vi "graficos3.vi"() -> ()   [LabVIEW 2019]
panel:
  out "Waveform Graph 3":cluster{dbl[]}[](graph)
  out "Waveform Graph 2":cluster{dbl, dbl, dbl[]}(graph)
  out "Waveform Chart 4":waveform(dbl)(graph)
  out "Waveform Chart 3":cluster{dbl, "Slide":dbl}(graph)
  out "Waveform Chart 2":dbl[](graph)
  out "Waveform Graph":dbl[](graph)
  out "Waveform Chart":dbl(graph)
  in  "stop":bool
  in  "Slide":dbl(slide) scale=0.0..50.0
  out "Thermometer":dbl(slide) scale=0.0..50.0
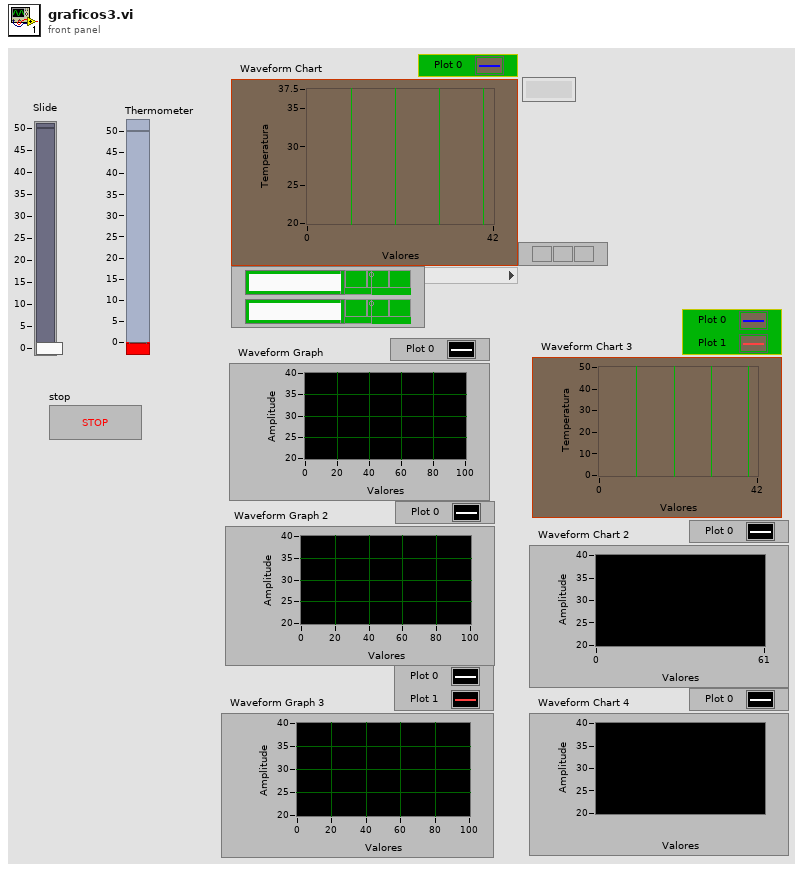
[diagram p1: front panel]
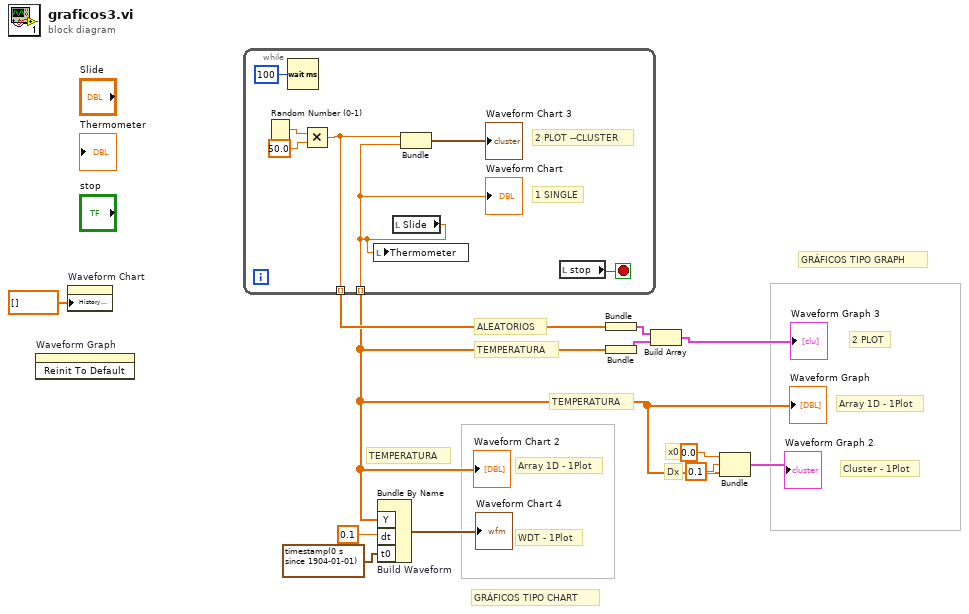
[diagram p0: block diagram]
diagram:
  # "GRÁFICOS TIPO CHART"
  # "GRÁFICOS TIPO GRAPH"
  # "ALEATORIOS"
  # "TEMPERATURA"
  # "TEMPERATURA"
  # "TEMPERATURA"
  # "Array 1D - 1Plot"
  # "Cluster - 1Plot"
  # "Dx"
  # "x0"
  # "2 PLOT"
  # "WDT - 1Plot"
  # "Array 1D - 1Plot"
  n1 = invoke on="Waveform Graph" class="WFGraph (strict)" method="Reinit To Default"() -> ()  [unwired: 3 in, 3 out]
  n2 = property on="Waveform Chart" class="WFChart (strict)"("History Data"=dbl[] []) -> ()  [unwired: 2 in, 2 out]
  n3 = while {
    tunnel: [w13] -> w1 mode=indexing
    tunnel: [w15] -> w5 mode=indexing
    stop <- w18 stop-if-true
    # "1 SINGLE"
    # "2 PLOT --CLUSTER"
    n4 = Random Number (0-1)() -> (number: 0 to 1=w17:dbl)
    n5 = Wait (ms)(milliseconds to wait=u32 100) -> ()  [unwired: 1 out]
    n6 = Multiply(x=w17, y=50.0) -> (x*y=w15:dbl)
    n7 = local read "Slide"() -> (w13:dbl)
    "Waveform Chart" <- w13
    n8 = local write "Thermometer"(w13) -> ()
    n9 = Bundle "Bundle"(w15, "Slide"=w13) -> (→"Waveform Chart 3":cluster{dbl, "Slide":dbl})  [unwired: 1 in]
    n10 = local read "stop"() -> (w18:bool)
  }
  "Waveform Graph" <- w1
  "Waveform Chart 2" <- w1
  n11 = Bundle By Name "Build Waveform"("Y"=w1, "dt"=0.1, "t0"=timestamp(0 s since 1904-01-01)) -> (→"Waveform Chart 4":waveform(dbl))  [unwired: 1 in]
  n12 = Bundle "Bundle"(w5) -> (w4:cluster{dbl[]})  [unwired: 1 in]
  n13 = Bundle(w1) -> (w3:cluster{dbl[]})  [unwired: 1 in]
  n14 = Build Array "Build Array"(w4, w3) -> (→"Waveform Graph 3":cluster{dbl[]}[])
  n15 = Bundle "Bundle"(0.0, 0.1, w1) -> (→"Waveform Graph 2":cluster{dbl, dbl, dbl[]})  [unwired: 1 in]
